vi "Matches.vi"(8 "error in (no error)":errorcluster, 10 "Actual":variant, 11 "LogicalNot in":refnum<class "LogicalNot.lvclass">) -> (0 "error out":errorcluster, 2 "Result":bool, 3 "LogicalNot out":refnum<class "LogicalNot.lvclass">)   [LabVIEW 2017, in "Constraint.lvlib" / "LogicalNot.lvclass"]
doc: "Evaluates the constraint for <B>Actual</B>. Returns true if the constraint is met."
uses:
  LogicalNot.lvclass
  UnaryOperator/UnaryOperator.lvclass
  Constraint/Constraint.lvclass
  C:/Users/de200256/Code/neuperger/lvunit/Constraint/UnaryOperator/UnaryOperator.lvclass
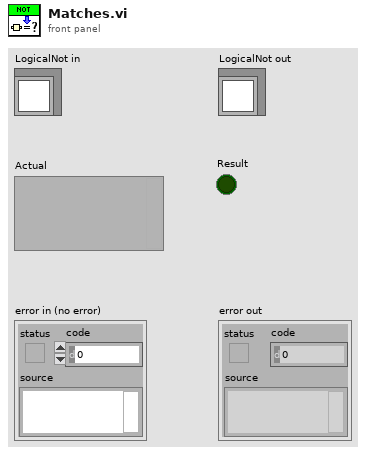
[diagram p1: front panel]
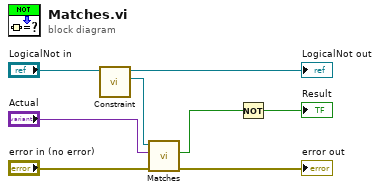
[diagram p0: block diagram]
diagram:
  n1 = call "Constraint.vi"("UnaryOperator in"="LogicalNot in") -> ("Constraint.lvlib:Constraint.lvclass"=w5:refnum<class "Constraint.lvclass">, "UnaryOperator out"=→"LogicalNot out":refnum<class "LogicalNot.lvclass">)  [unwired: 9 in]
  n2 = call-dynamic "Matches.vi"("error in (no error)"="error in (no error)", "Actual"="Actual", "Constraint in"=w5) -> ("error out"=→"error out":errorcluster, "Result"=w3:bool)  [unwired: 6 in, 1 out]
  n3 = Not(x=w3) -> (.not. x?=→"Result":bool)
